vi "DEMO.vi"() -> ()   [LabVIEW 2011]
uses:
  ScreenClass/Screen.lvclass
panel:
  out "error out":errorcluster caption="错误输出"
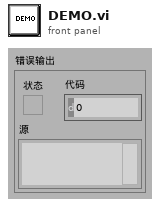
[diagram p1: front panel]
types:
  T1 = enum16{"PNG", "TIFF", "EMF", "JPEG", "BMP", "GIF"}
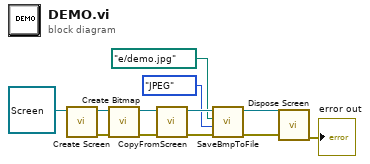
[diagram p0: block diagram]
diagram:
  n1 = call "Create Screen.vi"("Screen 输入"=refnum<class "Screen.lvclass"> refnum ("Screen.lvclass")) -> ("error out"=w10:errorcluster, "Screen 输出"=w11:refnum<class "Screen.lvclass">)  [unwired: 9 in]
  n2 = call "Create Bitmap.vi"("error in (no error)"=w10, "Screen 输入"=w11) -> ("error out"=w8:errorcluster, "Screen 输出"=w9:refnum<class "Screen.lvclass">)  [unwired: 8 in]
  n3 = call "CopyFromScreen.vi"("error in (no error)"=w8, "Screen 输入"=w9) -> ("error out"=w6:errorcluster, "Screen 输出"=w7:refnum<class "Screen.lvclass">)  [unwired: 8 in]
  n4 = call "SaveBmpToFile.vi"("error in (no error)"=w6, "文件格式"=T1."JPEG", "路径"=path "e:/demo.jpg", "Screen 输入"=w7) -> ("error out"=w2:errorcluster, "Screen 输出"=w3:refnum<class "Screen.lvclass">)  [unwired: 6 in]
  n5 = call "Dispose Screen.vi"("error in (no error)"=w2, "Screen 输入"=w3) -> ("error out"=→"error out":errorcluster)  [unwired: 8 in, 1 out]
